vi "Generate Build UEMessage.vi"(8 "Error In":errorcluster, 10 "Message":string, 11 "Project Build Tools in":refnum<class "Project Build Tools.lvclass">) -> (0 "Error Out":errorcluster, 3 "Project Build Tools out":refnum<class "Project Build Tools.lvclass">)   [LabVIEW 2019, in "Project Build Tools.lvclass"]
uses:
  Project Build Tools.lvclass
  Project Build Tools.lvclass/Project Build Tools.ctl
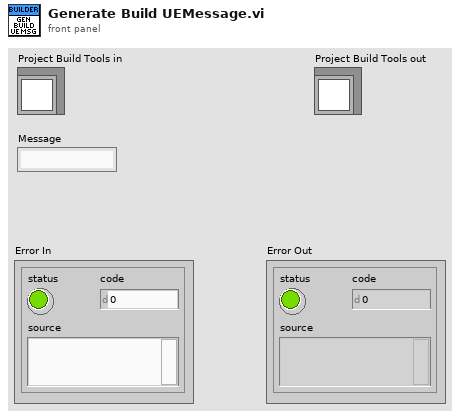
[diagram p1: front panel]
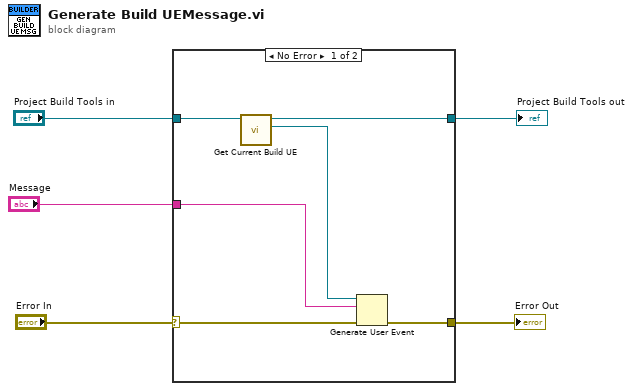
[diagram p0: block diagram]
diagram:
  n1 = case shown="No Error" "Error In" {
    selector: "Error In" -> [w8 w12]
    tunnel: [w11 w13] -> w5
    tunnel: "Project Build Tools in" -> [w9 w13]
    tunnel: "Message" -> [w7 _]
    tunnel: [w6 w12] -> w1
    frame No Error {
      n2 = call "Get Current Build UE.vi"("CD Build Tools in"=w9) -> ("Current Build UE"=w10:refnum<user-event>, "CD Build Tools out"=w11:refnum<class "Project Build Tools.lvclass">)  [unwired: 9 in]
      n3 = Generate User Event(user event=w10, event data cluster=w7, error in=w8) -> (error out=w6:errorcluster)  [unwired: 1 in, 1 out]
    }
    frame Error {
    }
  }
  "Project Build Tools out" <- w5
  "Error Out" <- w1
